vi "meth.PushArgs.vi"(0 "class.GLue in":refnum<class "class.GLue.lvclass">, 11 "error in (no error)":errorcluster, 13 "Variant in":variant) -> (4 "class.GLue out":refnum<class "class.GLue.lvclass">, 8 "NumArgs":i32, 15 "error out":errorcluster)   [LabVIEW 2014, in "GLue.lvlib" / "class.GLue.lvclass"]
uses:
  class.GLue.lvclass
  class.GLue.lvclass/class.GLue.ctl
  wrap.PushBool.vi
  wrap.PushString.vi
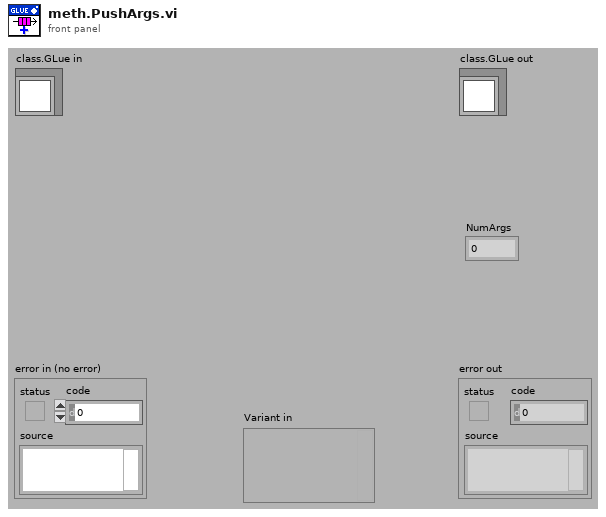
[diagram p1: front panel]
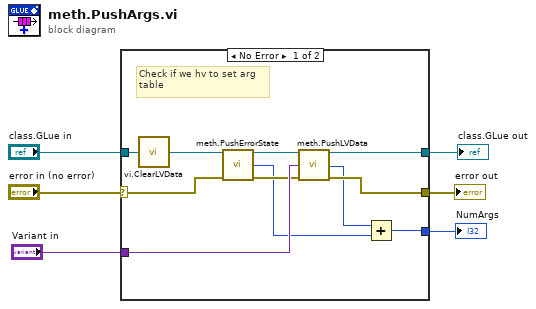
[diagram p0: block diagram]
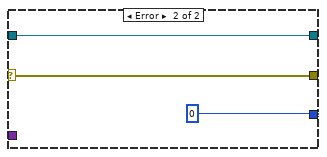
[diagram p2: hidden frame]
diagram:
  n1 = case shown="No Error" "error in (no error)" {
    selector: "error in (no error)" -> [w11 w20]
    tunnel: [w14 w20] -> w5
    tunnel: [w15 w19] -> w3
    tunnel: "class.GLue in" -> [w17 w19]
    tunnel: [w13 0] -> w2
    tunnel: "Variant in" -> [w16 _]
    frame No Error {
      # "Check if we hv to set arg\ntable"
      n2 = call "vi.ClearLVData.vi"("class.GLue in"=w17) -> ("class.GLue out"=w12:refnum<class "class.GLue.lvclass">)  [unwired: 14 in]
      n3 = call "meth.PushErrorState.vi"("class.GLue in"=w12, "error in (no error)"=w11) -> ("class.GLue out"=w9:refnum<class "class.GLue.lvclass">, "NumPushed"=w8:i32, "error out"=w10:errorcluster)  [unwired: 11 in]
      n4 = call "meth.PushLVData.vi"("class.GLue in"=w9, "variant in"=w16, "error in (no error)"=w10) -> ("class.GLue out"=w15:refnum<class "class.GLue.lvclass">, "NumPushed"=w7:i32, "error out"=w14:errorcluster)  [unwired: 10 in]
      n5 = Add(x=w7, y=w8) -> (x+y=w13:i32)
    }
    frame Error {
    }
  }
  "error out" <- w5
  "class.GLue out" <- w3
  "NumArgs" <- w2
